vi "层叠式顺序结构.vi"() -> ()   [LabVIEW 2018]
panel:
  out "数值 4":dbl
  in  "数值 3":dbl
  out "数值 2":dbl
  in  "数值":dbl
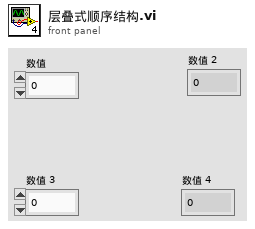
[diagram p1: front panel]
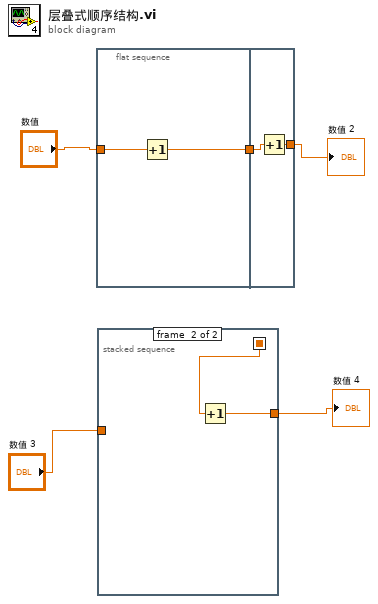
[diagram p0: block diagram]
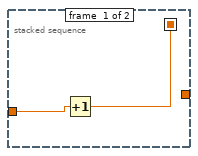
[diagram p2: hidden frame]
diagram:
  n1 = flat-sequence {
    tunnel: "数值" -> [w7]
    tunnel: [w6] -> w4
    tunnel: w4 -> [w9]
    tunnel: [w8] -> w3
    frame #0 {
      n2 = Increment(x=w7) -> (x+1=w6:dbl)
    }
    frame #1 {
      n3 = Increment(x=w9) -> (x+1=w8:dbl)
    }
  }
  n4 = stacked-sequence {
    seq-local: [w10 _] -> [_ w13]
    tunnel: "数值 3" -> [w11 _]
    tunnel: [_ w12] -> w1
    frame #0 {
      n5 = Increment(x=w11) -> (x+1=w10:dbl)
    }
    frame #1 {
      n6 = Increment(x=w13) -> (x+1=w12:dbl)
    }
  }
  "数值 4" <- w1
  "数值 2" <- w3
